vi "Get Path.vi"(11 "Base jettl in":refnum<class "Base jettl.lvclass">) -> (2 "Path":path)   [LabVIEW 2021, in "jettl.lvlib" / "Base jettl.lvclass"]
uses:
  Base jettl.lvclass
  Base jettl.lvclass/Base jettl.ctl
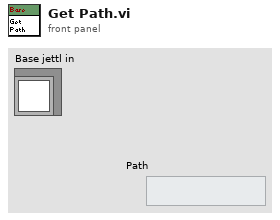
[diagram p1: front panel]
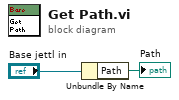
[diagram p0: block diagram]
diagram:
  n1 = Unbundle By Name("Base jettl in") -> ("Path"=→"Path":path)
